vi "Data Access.vi"(9 "Time Out In ms":i32=-1, 11 "Circular Buffer 2D U16 DVR Queue Circular Buffer in":refnum<class "Circular Buffer 2D U16 DVR Queue Circular Buffer.lvclass">) -> (1 "Time Out":bool, 2 "Data Out":u16[][](array[numeric]), 3 "Circular Buffer 2D U16 DVR Queue Circular Buffer out":refnum<class "Circular Buffer 2D U16 DVR Queue Circular Buffer.lvclass">)   [LabVIEW 2024, in "Circular Buffer 2D U16 DVR Queue Circular Buffer.lvclass"]
uses:
  Circular Buffer 2D U16 DVR Queue Circular Buffer.lvclass
  Circular Buffer 2D U16 DVR Queue Circular Buffer.lvclass/Circular Buffer 2D U16 DVR Queue Circular Buffer.ctl
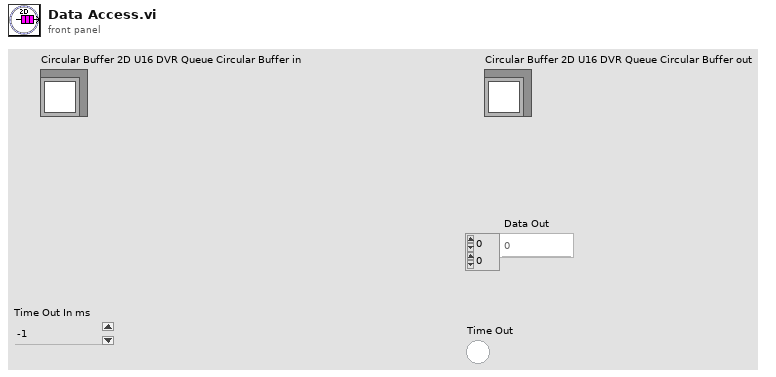
[diagram p1: front panel]
types:
  T1 = typedef "2D U16 DVR Queue.ctl" = refnum<queue>
  T2 = typedef "2D U16 DVR.ctl" = refnum<data-value>
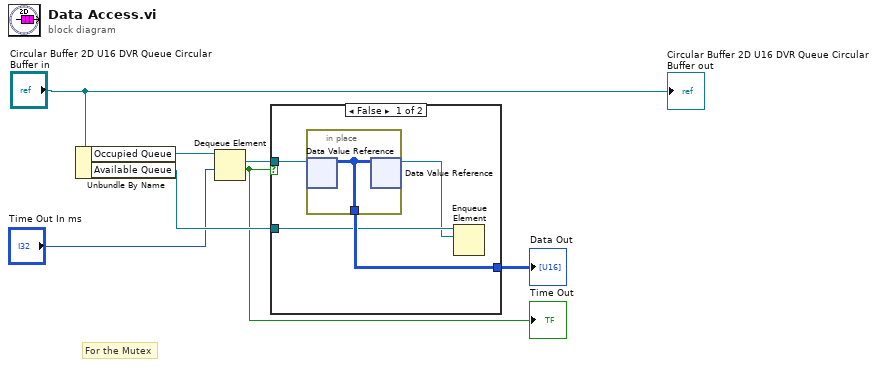
[diagram p0: block diagram]
diagram:
  # "For the Mutex"
  n1 = Unbundle By Name("Circular Buffer 2D U16 DVR Queue Circular Buffer in") -> ("Occupied Queue"=w6:T1, "Available Queue"=w4:T1)
  n2 = Dequeue Element(queue=w6, timeout in ms (-1)="Time Out In ms") -> (element=w5:T2, timed out?=w3:bool)  [unwired: 1 in, 2 out]
  "Time Out" <- w3
  n3 = case shown="False" w3 {
    tunnel: [w11 _] -> w7
    tunnel: w5 -> [w10 _]
    tunnel: w4 -> [w9 _]
    frame False {
      n4 = in-place {
        in-place-border: [w12] -> w11
        n5 = in-place-dvr #1(w10) -> (w12:u16[][])  [unwired: 1 out]
        n6 = in-place-dvr #1(w12) -> (w8:T2)  [unwired: 1 out]
      }
      n7 = Enqueue Element(queue=w9, element=w8) -> ()  [unwired: 2 in, 3 out]
    }
    frame True {
    }
  }
  "Data Out" <- w7
  "Circular Buffer 2D U16 DVR Queue Circular Buffer out" <- "Circular Buffer 2D U16 DVR Queue Circular Buffer in"
